vi "Build Channel List Dual Channel.vi"(9 "Channel":string, 10 "Data line":u16, 11 "Protocol capture resource name":string) -> (3 "String":string)   [LabVIEW 2021, in "Audio ADC Shared.lvlib"]
uses:
  Audio ADC Shared.lvlib
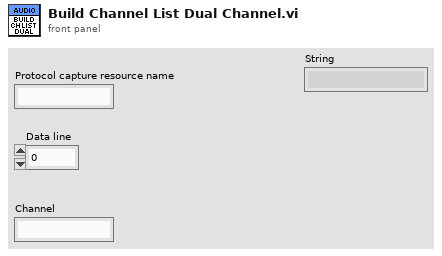
[diagram p1: front panel]
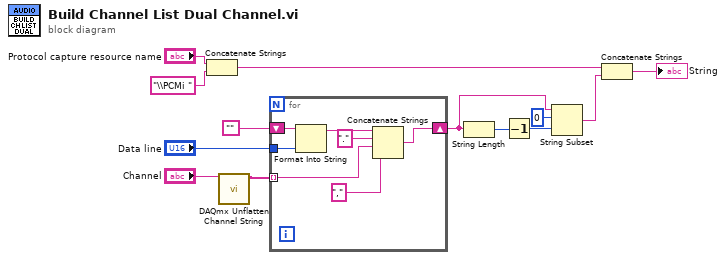
[diagram p0: block diagram]
diagram:
  n1 = Concatenate Strings("Protocol capture resource name", "\\PCMi " ("string")) -> (w11:string)
  n2 = call <vilib>:"DAQmx Unflatten Channel String.vi"("names in"="Channel") -> ("names out"=w10:string[])  [unwired: 13 in, 1 out]
  n3 = for {
    tunnel: "Data line" -> [w20]
    tunnel: w10 -> [w16] mode=indexing
    shift-right: [w14] -> w1
    shift-left: "" -> [w19]
    n4 = Format Into String(initial string=w19, w20) -> (resulting string=w18:string)  [unwired: 2 in, 1 out]
    n5 = Concatenate Strings(w18, "." ("string"), w16, "," ("string")) -> (w14:string)
  }
  n6 = String Length(string=w1) -> (length=w8:i32)
  n7 = Decrement(x=w8) -> (x-1=w7:i32)
  n8 = String Subset(string=w1, offset (0)=0, length (rest)=w7) -> (substring=w3:string)
  n9 = Concatenate Strings(w11, w3) -> (→"String":string)
